vi "_WriteSubData_TDMS_PWR.vi"(8 "error in (no error)":errorcluster, 10 "Sub Data in":T1 {"Control"."motor_ctrl_array"."sensor" format="%#.2f"; "Control"."motor_ctrl_array"."setpoint" format="%#.2f"; "Control"."dac_outputs" format="%#.2f"; "PWR"."motor_array"."motor_name" items=["Motor1", "Motor2", "Motor3", "Motor4", "Motor5", "Motor6"]}, 11 "Refnum in":refnum<k34>) -> (0 "error out":errorcluster, 3 "Refnum out":refnum<k34>)   [LabVIEW 2018]
uses:
  TypeDefsSubsea/Sub Data.ctl
  TypeDefsSubsea/Sub Status.ctl
  Shared/Type Defs/ROV States.ctl
  Shared/Type Defs/SMP.ctl
  Shared/Type Defs/PWR.ctl
  Shared/Type Defs/Motor.ctl
  Shared/Type Defs/MotorNames.ctl
  Shared/Type Defs/SmartCard.ctl
  Shared/Type Defs/Box Names.ctl
  TypeDefsSubsea/Sub Control.ctl
  TypeDefsSubsea/Modos Control.ctl
  TypeDefsSubsea/ROV Outputs.ctl
  TypeDefsSubsea/Motor Control.ctl
  TypeDefsSubsea/Type Defs Subsea.lvlib
  TypeDefsTopside/Type Defs Topside.lvlib
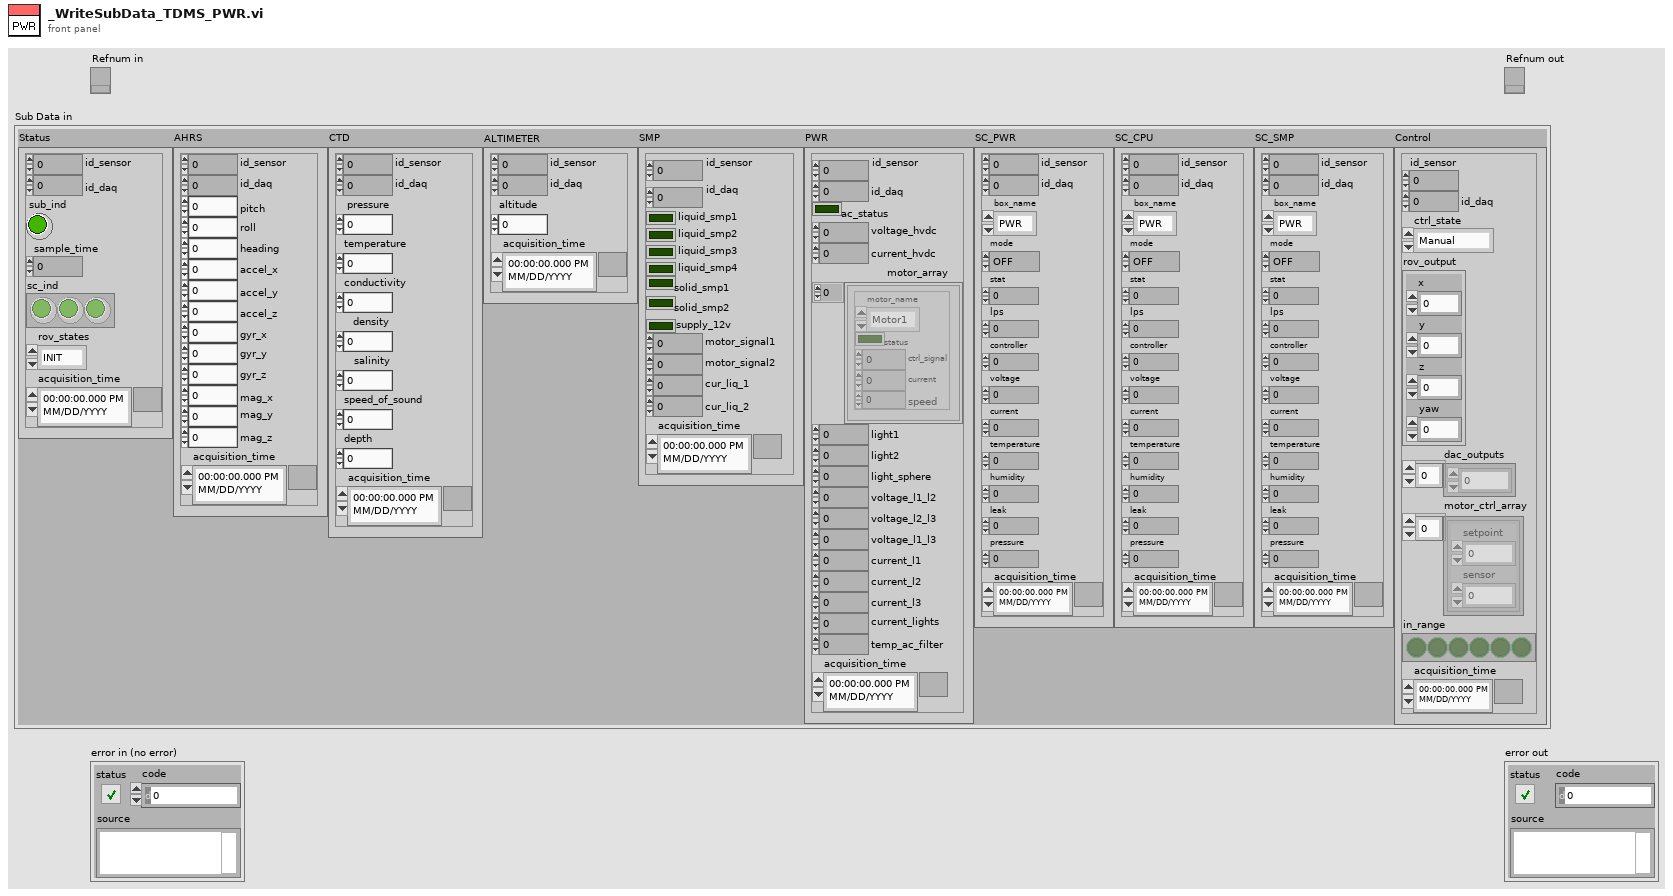
[diagram p1: front panel]
types:
  T1 = typedef "Type Defs Subsea.lvlib/Sub Data.ctl" = cluster{"Status":T2, "AHRS":cluster{"id_sensor":u32, "id_daq":u64, "pitch":dbl, "roll":dbl, "heading":dbl, "accel_x":dbl, "accel_y":dbl, "accel_z":dbl, "gyr_x":dbl, "gyr_y":dbl, "gyr_z":dbl, "mag_x":dbl, "mag_y":dbl, "mag_z":dbl, "acquisition_time":timestamp}, "CTD":cluster{"id_sensor":u32, "id_daq":u64, "pressure":dbl, "temperature":dbl, "conductivity":dbl, "density":dbl, "salinity":dbl, "speed_of_sound":dbl, "depth":dbl, "acquisition_time":timestamp}, "ALTIMETER":cluster{"id_sensor":u32, "id_daq":u64, "altitude":dbl, "acquisition_time":timestamp}, "SMP":T4, "PWR":T5, "SC_PWR":T8, "SC_CPU":T8, "SC_SMP":T8, "Control":T10}
  T2 = typedef "Type Defs Subsea.lvlib/Sub Status.ctl" = cluster{"id_sensor":u32, "id_daq":u32, "sub_ind":bool, "sample_time":i64, "sc_ind":bool[], "rov_states":T3, "acquisition_time":timestamp}
  T3 = typedef "Type Defs Subsea.lvlib/ROV States.ctl" = enum16{"INIT", "IDLE", "TEST", "RUN", "EMERGENCY", "EXIT"}
  T4 = typedef "Type Defs Subsea.lvlib/SMP.ctl" = cluster{"id_sensor":u32, "id_daq":u64, "liquid_smp1":bool, "liquid_smp2":bool, "liquid_smp3":bool, "liquid_smp4":bool, "solid_smp1":bool, "solid_smp2":bool, "supply_12v":bool, "motor_signal1":dbl, "motor_signal2":dbl, "cur_liq_1":dbl, "cur_liq_2":dbl, "acquisition_time":timestamp}
  T5 = typedef "Type Defs Topside.lvlib/PWR.ctl" = cluster{"id_sensor":u32, "id_daq":u64, "ac_status":bool, "voltage_hvdc":dbl, "current_hvdc":dbl, "motor_array":T6[], "light1":dbl, "light2":dbl, "light_sphere":dbl, "voltage_l1_l2":dbl, "voltage_l2_l3":dbl, "voltage_l1_l3":dbl, "current_l1":dbl, "current_l2":dbl, "current_l3":dbl, "current_lights":dbl, "temp_ac_filter":dbl, "acquisition_time":timestamp}
  T6 = typedef "Type Defs Subsea.lvlib/Motor.ctl" = cluster{"motor_name":T7, "status":bool, "ctrl_signal":dbl, "current":dbl, "speed":dbl}
  T7 = typedef "Type Defs Subsea.lvlib/MotorNames.ctl" = u16
  T8 = typedef "Type Defs Subsea.lvlib/SmartCard.ctl" = cluster{"id_sensor":u32, "id_daq":u64, "box_name":T9, "mode":enum16{"OFF", "STANDBY", "TESTING", "RUN", "EMERGENCY"}, "stat":dbl, "lps":dbl, "controller":dbl, "voltage":dbl, "current":dbl, "temperature":dbl, "humidity":dbl, "leak":dbl, "pressure":dbl, "acquisition_time":timestamp}
  T9 = typedef "Type Defs Subsea.lvlib/Box Names.ctl" = enum16{"PWR", "CPU", "SMP"}
  T10 = typedef "Type Defs Subsea.lvlib/Sub Control.ctl" = cluster{"id_sensor":u32, "id_daq":u64, "ctrl_state":T11, "rov_output":T12, "dac_outputs":dbl[], "motor_ctrl_array":T13[], "in_range":bool[], "acquisition_time":timestamp}
  T11 = typedef "Type Defs Subsea.lvlib/Modos Control.ctl" = enum16{"Manual", "Profundidad", "Altitud", "Rumbo", "P+R"}
  T12 = typedef "Type Defs Subsea.lvlib/ROV Outputs.ctl" = cluster{"x":dbl, "y":dbl, "z":dbl, "yaw":dbl}
  T13 = typedef "Type Defs Subsea.lvlib/Motor Control.ctl" = cluster{"setpoint":dbl, "sensor":dbl}
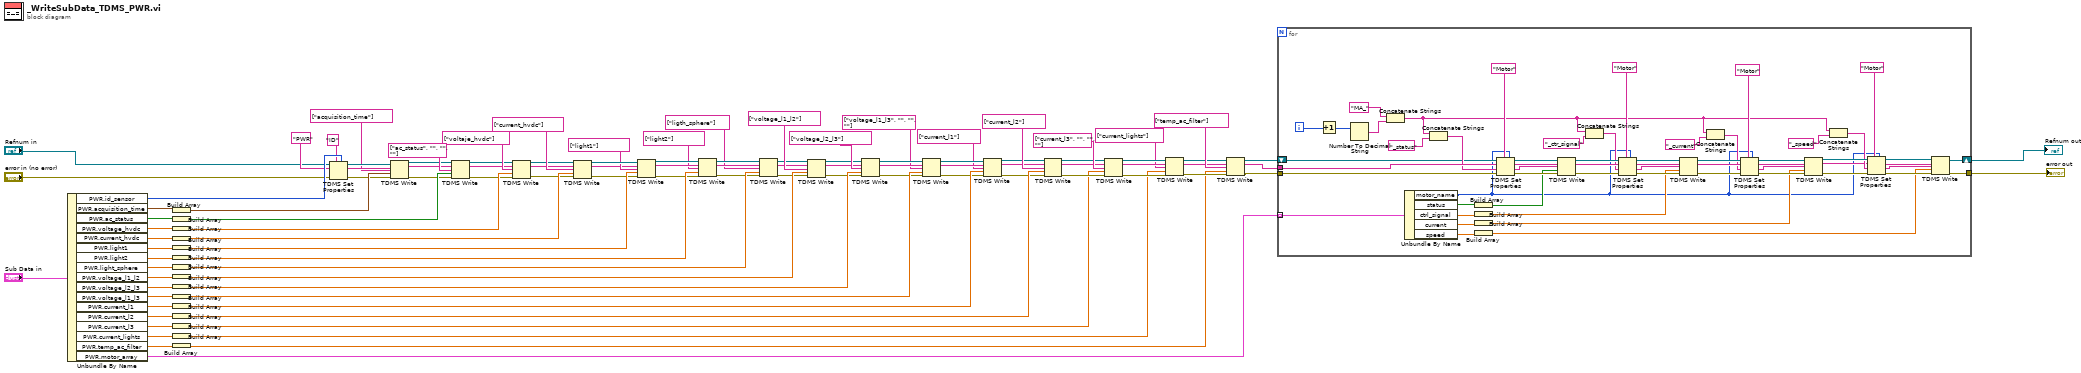
[diagram p0: block diagram]
diagram:
  n1 = Unbundle By Name("Sub Data in") -> ("PWR.id_sensor"=w88:u32, "PWR.acquisition_time"=w89:timestamp, "PWR.ac_status"=w90:bool, "PWR.voltage_hvdc"=w39:dbl, "PWR.current_hvdc"=w38:dbl, "PWR.light1"=w37:dbl, "PWR.light2"=w36:dbl, "PWR.light_sphere"=w35:dbl, "PWR.voltage_l1_l2"=w34:dbl, "PWR.voltage_l2_l3"=w33:dbl, "PWR.voltage_l1_l3"=w32:dbl, "PWR.current_l1"=w31:dbl, "PWR.current_l2"=w30:dbl, "PWR.current_l3"=w17:dbl, "PWR.current_lights"=w16:dbl, "PWR.temp_ac_filter"=w15:dbl, "PWR.motor_array"=w6:T6[])
  n2 = Build Array(w89) -> (w91:timestamp[])
  n3 = Build Array(w90) -> (w92:bool[])
  n4 = Build Array(w39) -> (w93:dbl[])
  n5 = Build Array(w38) -> (w94:dbl[])
  n6 = Build Array(w37) -> (w95:dbl[])
  n7 = Build Array(w36) -> (w96:dbl[])
  n8 = Build Array(w35) -> (w97:dbl[])
  n9 = Build Array(w34) -> (w98:dbl[])
  n10 = Build Array(w33) -> (w99:dbl[])
  n11 = Build Array(w32) -> (w100:dbl[])
  n12 = Build Array(w31) -> (w101:dbl[])
  n13 = Build Array(w30) -> (w102:dbl[])
  n14 = Build Array(w17) -> (w14:dbl[])
  n15 = Build Array(w16) -> (w13:dbl[])
  n16 = Build Array(w15) -> (w12:dbl[])
  n17 = TDMS Set Properties(5:w88, 7:"ID" ("property names"), 8:"error in (no error)", 10:"PWR" ("group name in (Untitled)"), 11:"Refnum in") -> (0:w51:errorcluster, 2:w50:string, 3:w48:refnum<k34>)  [unwired: 1 in, 1 out]
  n18 = TDMS Write(0:w48, 5:w50, 7:string[] ["acquisition_time"] ("channel name(s) in (Untitled)"), 9:w91, 11:w51) -> (4:w44:refnum<k34>, 6:w43:string, 15:w45:errorcluster)  [unwired: 1 in, 1 out]
  n19 = TDMS Write(0:w44, 5:w43, 7:string[] ["ac_status", "", "", ""] ("channel name(s) in (Untitled)"), 9:w92, 11:w45) -> (4:w56:refnum<k34>, 6:w55:string, 15:w57:errorcluster)  [unwired: 1 in, 1 out]
  n20 = TDMS Write(0:w56, 5:w55, 7:string[] ["voltaje_hvdc"] ("channel name(s) in (Untitled)"), 9:w93, 11:w57) -> (4:w53:refnum<k34>, 6:w52:string, 15:w54:errorcluster)  [unwired: 1 in, 1 out]
  n21 = TDMS Write(0:w53, 5:w52, 7:string[] ["current_hvdc"] ("channel name(s) in (Untitled)"), 9:w94, 11:w54) -> (4:w10:refnum<k34>, 6:w8:string, 15:w11:errorcluster)  [unwired: 1 in, 1 out]
  n22 = TDMS Write(0:w10, 5:w8, 7:string[] ["light1"] ("channel name(s) in (Untitled)"), 9:w95, 11:w11) -> (4:w63:refnum<k34>, 6:w64:string, 15:w62:errorcluster)  [unwired: 1 in, 1 out]
  n23 = TDMS Write(0:w63, 5:w64, 7:string[] ["light2"] ("channel name(s) in (Untitled)"), 9:w96, 11:w62) -> (4:w66:refnum<k34>, 6:w67:string, 15:w65:errorcluster)  [unwired: 1 in, 1 out]
  n24 = TDMS Write(0:w66, 5:w67, 7:string[] ["ligth_sphere"] ("channel name(s) in (Untitled)"), 9:w97, 11:w65) -> (4:w82:refnum<k34>, 6:w84:string, 15:w83:errorcluster)  [unwired: 1 in, 1 out]
  n25 = TDMS Write(0:w82, 5:w84, 7:string[] ["voltage_l1_l2"] ("channel name(s) in (Untitled)"), 9:w98, 11:w83) -> (4:w79:refnum<k34>, 6:w80:string, 15:w85:errorcluster)  [unwired: 1 in, 1 out]
  n26 = TDMS Write(0:w79, 5:w80, 7:string[] ["voltage_l2_l3"] ("channel name(s) in (Untitled)"), 9:w99, 11:w85) -> (4:w77:refnum<k34>, 6:w78:string, 15:w76:errorcluster)  [unwired: 1 in, 1 out]
  n27 = TDMS Write(0:w77, 5:w78, 7:string[] ["voltage_l1_l3", "", "", ""] ("channel name(s) in (Untitled)"), 9:w100, 11:w76) -> (4:w70:refnum<k34>, 6:w71:string, 15:w69:errorcluster)  [unwired: 1 in, 1 out]
  n28 = TDMS Write(0:w70, 5:w71, 7:string[] ["current_l1"] ("channel name(s) in (Untitled)"), 9:w101, 11:w69) -> (4:w73:refnum<k34>, 6:w74:string, 15:w72:errorcluster)  [unwired: 1 in, 1 out]
  n29 = TDMS Write(0:w73, 5:w74, 7:string[] ["current_l2"] ("channel name(s) in (Untitled)"), 9:w102, 11:w72) -> (4:w19:refnum<k34>, 6:w7:string, 15:w18:errorcluster)  [unwired: 1 in, 1 out]
  n30 = TDMS Write(0:w19, 5:w7, 7:string[] ["current_l3", "", "", ""] ("channel name(s) in (Untitled)"), 9:w14, 11:w18) -> (4:w22:refnum<k34>, 6:w23:string, 15:w21:errorcluster)  [unwired: 1 in, 1 out]
  n31 = TDMS Write(0:w22, 5:w23, 7:string[] ["current_lights"] ("channel name(s) in (Untitled)"), 9:w13, 11:w21) -> (4:w25:refnum<k34>, 6:w26:string, 15:w24:errorcluster)  [unwired: 1 in, 1 out]
  n32 = TDMS Write(0:w25, 5:w26, 7:string[] ["temp_ac_filter"] ("channel name(s) in (Untitled)"), 9:w12, 11:w24) -> (4:w3:refnum<k34>, 6:w4:string, 15:w5:errorcluster)  [unwired: 1 in, 1 out]
  n33 = for {
    tunnel: w6 -> [w148] mode=indexing
    tunnel: w5 -> [w143]
    tunnel: w4 -> [w142]
    shift-right: [w106] -> w1
    shift-left: w3 -> [w105]
    tunnel: [w104] -> w2
    i -> [w146]
    n34 = Increment(x=w146) -> (x+1=w147:i32)
    n35 = Number To Decimal String(number=w147) -> (decimal integer string=w144:string)  [unwired: 1 in]
    n36 = Concatenate Strings("MA_" ("string"), w144) -> (w111:string)
    n37 = Unbundle By Name(w148) -> ("motor_name"=w103:T7, "status"=w135:bool, "ctrl_signal"=w134:dbl, "current"=w133:dbl, "speed"=w132:dbl)
    n38 = Concatenate Strings(w111, "_status" ("string")) -> (w119:string)
    n39 = Build Array(w135) -> (w131:bool[])
    n40 = Build Array(w134) -> (w130:dbl[])
    n41 = Build Array(w133) -> (w129:dbl[])
    n42 = Build Array(w132) -> (w123:dbl[])
    n43 = TDMS Set Properties(5:w103, 7:"Motor" ("property names"), 8:w143, 9:w119, 10:w142, 11:w105) -> (0:w154:errorcluster, 1:w115:string, 2:w138:string, 3:w137:refnum<k34>)
    n44 = TDMS Write(0:w137, 5:w138, 7:w115, 9:w131, 11:w154) -> (4:w136:refnum<k34>, 6:w155:string, 15:w141:errorcluster)  [unwired: 1 in, 1 out]
    n45 = Concatenate Strings(w111, "_ctr_signal" ("string")) -> (w117:string)
    n46 = TDMS Set Properties(5:w103, 7:"Motor" ("property names"), 8:w141, 9:w117, 10:w155, 11:w136) -> (0:w149:errorcluster, 1:w116:string, 2:w151:string, 3:w150:refnum<k34>)
    n47 = TDMS Write(0:w150, 5:w151, 7:w116, 9:w130, 11:w149) -> (4:w152:refnum<k34>, 6:w153:string, 15:w140:errorcluster)  [unwired: 1 in, 1 out]
    n48 = Concatenate Strings(w111, "_current" ("string")) -> (w113:string)
    n49 = TDMS Set Properties(5:w103, 7:"Motor" ("property names"), 8:w140, 9:w113, 10:w153, 11:w152) -> (0:w157:errorcluster, 1:w112:string, 2:w159:string, 3:w158:refnum<k34>)
    n50 = TDMS Write(0:w158, 5:w159, 7:w112, 9:w129, 11:w157) -> (4:w124:refnum<k34>, 6:w107:string, 15:w125:errorcluster)  [unwired: 1 in, 1 out]
    n51 = Concatenate Strings(w111, "_speed" ("string")) -> (w109:string)
    n52 = TDMS Set Properties(5:w103, 7:"Motor" ("property names"), 8:w125, 9:w109, 10:w107, 11:w124) -> (0:w126:errorcluster, 1:w108:string, 2:w128:string, 3:w127:refnum<k34>)
    n53 = TDMS Write(0:w127, 5:w128, 7:w108, 9:w123, 11:w126) -> (4:w106:refnum<k34>, 15:w104:errorcluster)  [unwired: 1 in, 2 out]
  }
  "error out" <- w2
  "Refnum out" <- w1
